vi "Host Run 4 Wire xVDT Sim.vi"() -> ()   [LabVIEW 2010]
uses:
  <vilib>/userDefined/High Color/nirio_resource_hc.ctl
  <vilib>/rvi/interface/nirviOpenFPGA/nirviOpenFPGA.xnode
  FPGA Bitfiles/xVDTSimulation_7852_FPGA4WirexVDTSim_88E4B036.lvbitx
  FPGA/FPGA 4 Wire xVDT Sim.vi
  <vilib>/rvi/ClientSDK/nirviWhatTheDeviceIsDoing.ctl
  <vilib>/rvi/interface/nirviReadWriteControl/nirviReadWriteControl.xnode
  <vilib>/rvi/interface/common/niFpgaNodeNameForErrorReporting.ctl
  <vilib>/rvi/errors/niLvFpgaWhatHappensToTopLevelVI.ctl
  <vilib>/rvi/interface/nirviCloseFPGA/nirviCloseFPGA.xnode
  <vilib>/FPGAPlugInAG/PXI-7852R/niLvFpga_Open_PXI-7852R.vi
  <vilib>/Utility/error.llb/Error Cluster From Error Code.vi
  <vilib>/rvi/errors/niLvFpgaAdjustHostInterfaceError.vi
  <vilib>/FPGAPlugInAG/PXI-7852R/niLvFpga_Close_PXI-7852R.vi
  NiFpgaLv.dll
panel:
  out "Scaling Factor":fxp<+/-,19,5> format="%.16g"
  in  "Sensitivity (V/V/mm)":dbl=0.05
  out "error out":errorcluster
  in  "stop":bool
  in  "Position (mm)":dbl(slide) caption="Position" scale=-20.0..20.0 scale format="%.2f"
  # "Setup"
  # "Run-Time"
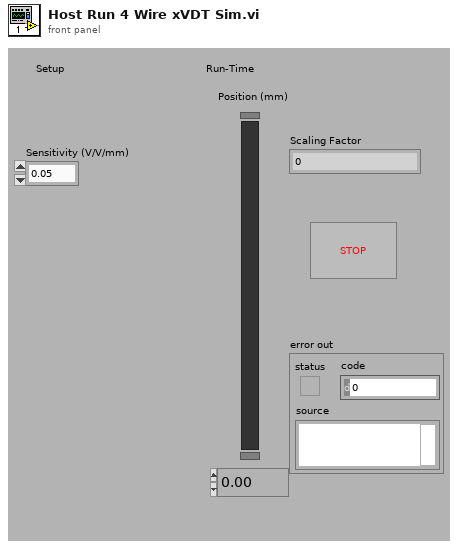
[diagram p1: front panel]
types:
  T1 = typedef "niFpgaNodeNameForErrorReporting.ctl" = enum16{"Open FPGA VI Reference", "Read/Write Control", "Invoke Method: Abort", "Invoke Method: Acknowledge IRQ", "Invoke Method: Download", "Invoke Method: FIFO.Configure", "Invoke Method: FIFO.Read", "Invoke Method: FIFO.Start", "Invoke Method: FIFO.Stop", "Invoke Method: FIFO.Write", "Invoke Method: Reset", "Invoke Method: Run", "Invoke Method: Wait on IRQ", "Close FPGA VI Reference"}
  T2 = typedef "niLvFpgaWhatHappensToTopLevelVI.ctl" = enum16{"top level VI scripted behind XNode", "top level VI inlined behind XNode"}
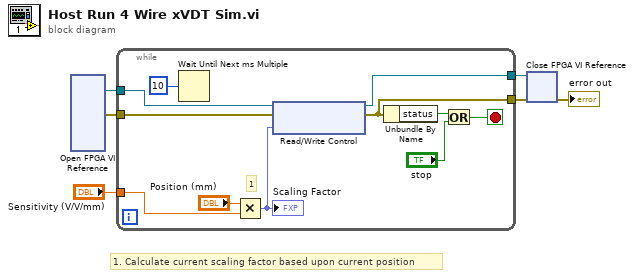
[diagram p0: block diagram]
diagram:
  # "1. Calculate current scaling factor based upon current position"
  n1 = xnode "Open FPGA VI Reference"() -> ("FPGA VI Reference Out"=w3:refnum<k20>, "error out"=w2:errorcluster)  [unwired: 2 in]
  n2 = while {
    tunnel: w2 -> [w8]
    tunnel: [w13] -> w6
    tunnel: "Sensitivity (V/V/mm)" -> [w12]
    tunnel: w3 -> [w9]
    tunnel: [w7] -> w1
    stop <- w15 stop-if-true
    # "1"
    n3 = Wait Until Next ms Multiple(millisecond multiple=u32 10) -> ()  [unwired: 1 out]
    n4 = Multiply(x="Position (mm)", y=w12) -> (x*y=w10:fxp<+/-,19,5>)
    "Scaling Factor" <- w10
    n5 = xnode "Read/Write Control"("FPGA VI Reference In"=w9, "error in"=w8, "Scaling Factor"=w10) -> ("FPGA VI Reference Out"=w7:refnum<k20>, "error out"=w13:errorcluster)
    n6 = Unbundle By Name(w13) -> ("status"=w14:bool)
    n7 = Or(x=w14, y="stop") -> (x .or. y?=w15:bool)
  }
  n8 = xnode "Close FPGA VI Reference"("FPGA VI Reference In"=w1, "error in"=w6) -> ("error out"=→"error out":errorcluster)
